vi "DecodeSubCar.vi"(8 "error in (no error)":errorcluster, 11 "ISO 14443 A UP in":refnum<class "ISO 14443 A UP.lvclass">) -> (0 "error out":errorcluster, 3 "ISO 14443 A UP out":refnum<class "ISO 14443 A UP.lvclass">)   [LabVIEW 2019, in "ISO 14443 A UP.lvclass"]
uses:
  ISO 14443 A UP.lvclass
  TypeDef/Store.ctl
  ISO 14443 A UP.lvclass/ISO 14443 A UP.ctl
  RFID system.lvclass
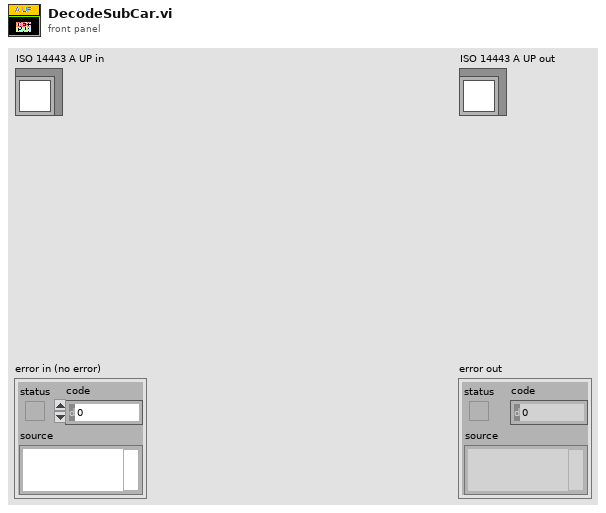
[diagram p1: front panel]
types:
  T1 = typedef "Store.ctl" = enum16{"envelope", "noise", "demSubCar", "CH_frame", "Decode", "demodulate", "in", "out", "sum", "subCarrier", "frame", "command", "encode", "modulate", "encode_UP", "modulate_up", "demod_up", "envelop_up", "sum_up", "out_up", "in_up"}
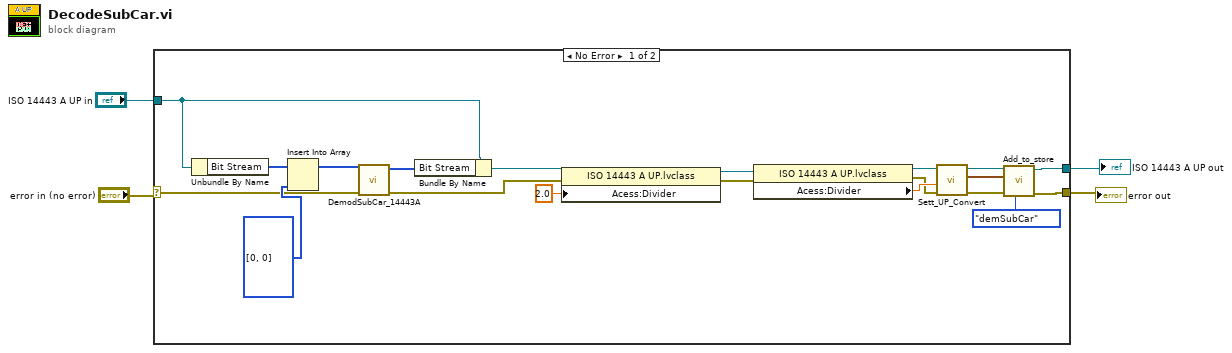
[diagram p0: block diagram]
diagram:
  n1 = case shown="No Error" "error in (no error)" {
    selector: "error in (no error)" -> [w14 w25]
    tunnel: [w15 w26] -> w2
    tunnel: "ISO 14443 A UP in" -> [w17 w26]
    tunnel: [w10 w25] -> w1
    frame No Error {
      n2 = Unbundle By Name(w17) -> ("Bit Stream"=w18:u8[])
      n3 = Insert Into Array(array=w18, new element=u8[] [0, 0]) -> (w23:u8[])  [unwired: 1 in]
      n4 = call "DemodSubCar_14443A.vi"("error in (no error)"=w14, "output array"=w23) -> ("error out"=w7:errorcluster, "Array"=w16:u8[])  [unwired: 8 in]
      n5 = Bundle By Name(cluster=w17, "Bit Stream"=w16) -> (w9:refnum<class "ISO 14443 A UP.lvclass">)
      n6 = property class="ISO 14443 A UP.lvclass"(reference=w9, error in=w7, "Acess:Divider"=2.0 ("Divider")) -> (reference out=w8:refnum<class "ISO 14443 A UP.lvclass">, error out=w6:errorcluster)
      n7 = property class="ISO 14443 A UP.lvclass"(reference=w8, error in=w6) -> (reference out=w13:refnum<class "ISO 14443 A UP.lvclass">, error out=w11:errorcluster, "Acess:Divider"=w12:dbl)
      n8 = call-dynamic "Sett_UP_Convert.vi"("error in (no error)"=w11, "Divider(1)"=w12, "ISO 14443 A UP in"=w13) -> ("error out"=w21:errorcluster, "Waveform"=w20:waveform(dbl), "ISO 14443 A UP out"=w22:refnum<class "ISO 14443 A UP.lvclass">)  [unwired: 6 in]
      n9 = call "Add_to_store.vi"("Store"=Store."demSubCar", "error in (no error)"=w21, "Waveform"=w20, "RFID system in"=w22) -> ("error out"=w10:errorcluster, "RFID system out"=w15:refnum<class "ISO 14443 A UP.lvclass">)  [unwired: 6 in]
    }
    frame Error {
    }
  }
  "error out" <- w1
  "ISO 14443 A UP out" <- w2
